vi "Array_Replace 2nd Row.vi"(8 "1 Row":string[][](array[string])=[["1231235", "0:04:10", "24", "24", "24", "24", "24", "040", "030.5", "077.5", "078.9", "048.5", "080.6", "040.000000E+0", "0.000000E+0", "0.000000E+0", "0.000000E+0", "0.000000E+0", "0.000000E+0", "038.700000E+0", "0", "0", "0", "0", "0", "0", "0178.200000E+36", "08.949600E+0", "05.292000E+0", "040531400E+0", "090900000E+0", "022.657000E+0", "040384600E+0", "01.566800E+0", "08.632800E+0", "000257200E+0", "01.950200E+0", "010932200E+0", "06.315200E+0", "050382800E+0", "04.250600E+0", "00.854800E+0"]], 9 "2 Rows":string[][](array[string])) -> (1 "Ouput Array":string[][](array[string]))   [LabVIEW 2009]
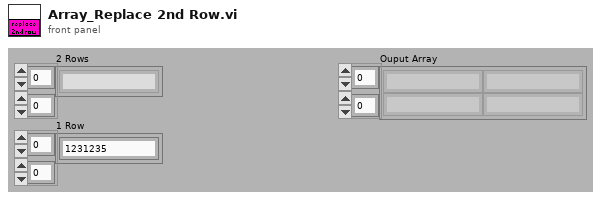
[diagram p1: front panel]
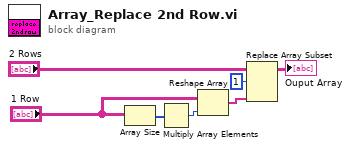
[diagram p0: block diagram]
diagram:
  n1 = Array Size(array="1 Row") -> (size(s)=w7:i32[])
  n2 = Multiply Array Elements(1:w7) -> (0:w6:i32)
  n3 = Reshape Array("1 Row", w6) -> (w4:string[])
  n4 = Replace Array Subset(array="2 Rows", new element=w4, index (row)=1) -> (→"Ouput Array":string[][])  [unwired: 1 in]
